vi "Bool Latch.vi"(9 "set":bool, 10 "value":bool) -> (2 "out":bool)   [LabVIEW 2015, in "Engine Simulation Toolkit.lvlib"]
uses:
  Engine Simulation Toolkit.lvlib
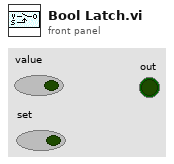
[diagram p1: front panel]
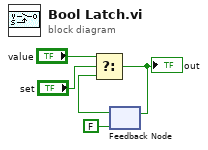
[diagram p0: block diagram]
diagram:
  n1 = feedback #1(FALSE) -> (w1:bool)
  n2 = Select(t="value", s="set", f=w1) -> (s? t:f=w2:bool)
  "out" <- w2
  n3 = feedback-in #1(w2) -> ()
